vi "REPORT_GEAR_save_pdf.vi"(8 "error_in":errorcluster) -> (0 "error_out":errorcluster)   [LabVIEW 2019]
uses:
  FGV/REPORTS_records_display/FGV_REPORTS_records_display.ctl
  typedef/REPORT_GEAR_all_info.ctl
  typedef/REPORT_GEAR_header_data_display.ctl
  typedef/REPORT_GEAR_statuses.ctl
  <vilib>/Exaprom PDF/Controls/Page Controls/Page setup.ctl
  <vilib>/Exaprom PDF/Controls/Page Controls/Page size.ctl
  <vilib>/Exaprom PDF/Controls/Page Controls/Page Orientation.ctl
  <vilib>/Exaprom PDF/Controls/Page Controls/Page Layout Custom.ctl
  <vilib>/Exaprom PDF/Controls/Page Controls/Page margins.ctl
  <vilib>/Exaprom PDF/Controls/Image Controls/Image alignment and position.ctl
  <vilib>/Exaprom PDF/Controls/Image Controls/Image aligment.ctl
  <vilib>/Exaprom PDF/Controls/Table Controls/Row Predefined borders cluster.ctl
  <vilib>/Exaprom PDF/Controls/Table Controls/Row Predefined borders.ctl
  <vilib>/Exaprom PDF/Controls/Table Controls/Cell Font, type, Alignment and LS V2.ctl
  <vilib>/Exaprom PDF/Controls/Table Controls/Cell Type, Alignment and LS.ctl
  <vilib>/Exaprom PDF/Controls/Table Controls/Cell Alignment 20px.ctl
  <vilib>/Exaprom PDF/Controls/Table Controls/Text vertical arrangement.ctl
  <vilib>/Exaprom PDF/Controls/Text Controls/Line spacing.ctl
  <vilib>/Exaprom PDF/Controls/Font Controls/Font complete cluster.ctl
  <vilib>/Exaprom PDF/Controls/Font Controls/Font size.ctl
  <vilib>/Exaprom PDF/Controls/Font Controls/Font color.ctl
  <vilib>/Exaprom PDF/Controls/Font Controls/Type and encoding.ctl
  <vilib>/Exaprom PDF/Controls/Text Controls/Unicode/Type and run direction.ctl
  REPORT_font_for_pdf_report.ctl
  _misc/AULocalize/SubVIs/Get Localized Phrase Compact Interface 0D.vi
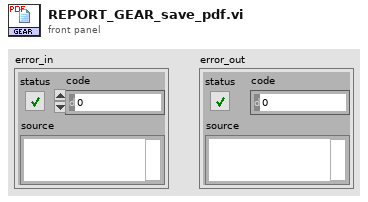
[diagram p1: front panel]
types:
  T1 = typedef "REPORT_GEAR_all_info.ctl" = cluster{"serial":string, "filter_OP":string, "REPORT_GEAR_header":T2, "operations":string[][], "operation_statuses":T3[], "results":string[][], "result_statuses":T3[], "batches":string[][], "batch_statuses":T3[], "column_headers":string[], "displayed_rows":string[][], "displayed_statuses":T3[], "column_widths":i16[]}
  T2 = typedef "REPORT_GEAR_header_data_display.ctl" = cluster{"ID":string, "creation_time":string, "last_station":string, "last_status":string, "pinion_serial":string, "batch_code":string}
  T3 = typedef "REPORT_GEAR_statuses.ctl" = enum16{"OP_OK_hide", "OP_OK_show", "OP_NOK_hide", "OP_NOK_show", "OP_interrupted_hide", "OP_interrupted_show", "OP_in_operation_hide", "OP_in_operation_show", "OP_unexpected_hide", "OP_unexpected_show", "RE_REAL_OK", "RE_REAL_NOK", "RE_STRING", "RE_sub_header", "RE_no_data", "RE_unexpected", "BA_sub_header", "BA_data", "BA_no_data"}
  T4 = typedef "FGV_REPORTS_records_display.ctl" = enum16{"initialize", "GEAR_set_serial", "GEAR_set_header", "GEAR_set_operations", "GEAR_set_results", "GEAR_set_batches", "GEAR_get_serial", "GEAR_get_operation_IDs", "GEAR_toggle_results", "GEAR_show_all_results", "GEAR_hide_all_results", "GEAR_display", "GEAR_filter", "GEAR_restore", "GEAR_clear", "GEAR_get_all_info", "DATES_set_dates", "DATES_set_gears", "DATES_display", "DATES_filter", "DATES_first_page", "DATES_previous_page", "DATES_next_page", "DATES_last_page", "DATES_restore", "DATES_clear", "DATES_get_all_info", "PBATCH_set_batch_no", "PBATCH_set_gears", "PBATCH_display", "PBATCH_filter", "PBATCH_first_page", "PBATCH_previous_page", "PBATCH_next_page", "PBATCH_last_page", "PBATCH_restore", "PBATCH_clear", "PBATCH_get_all_info", "OPRTN_set_OP", "OPRTN_set_dates", "OPRTN_set_gears", "OPRTN_set_hidden_columns", "OPRTN_display", "OPRTN_filter", "OPRTN_filter_no_page_reset", "OPRTN_first_page", "OPRTN_previous_page", "OPRTN_next_page", "OPRTN_last_page", "OPRTN_restore", "OPRTN_clear", "OPRTN_get_all_info", "CFG_set_type", "CFG_set_dates", "CFG_set_records", "CFG_display", "CFG_filter", "CFG_first_page", "CFG_previous_page", "CFG_next_page", "CFG_last_page", "CFG_restore", "CFG_clear", "CFG_get_all_info", "AUDIT_set_dates", "AUDIT_set_records", "AUDIT_display", "AUDIT_filter", "AUDIT_first_page", "AUDIT_previous_page", "AUDIT_next_page", "AUDIT_last_page", "AUDIT_restore", "AUDIT_clear", "AUDIT_get_all_info", "OKNOK_set_dates", "OKNOK_set_records", "OKNOK_display", "OKNOK_restore", "OKNOK_clear", "OKNOK_get_all_info", "REWORKS_set_dates", "REWORKS_set_from_to", "REWORKS_set_records", "REWORKS_display", "REWORKS_filter", "REWORKS_first_page", "REWORKS_previous_page", "REWORKS_next_page", "REWORKS_last_page", "REWORKS_restore", "REWORKS_clear", "REWORKS_get_all_info", "PACE_set_dates", "PACE_set_limits", "PACE_set_records", "PACE_display", "PACE_restore", "PACE_clear", "PACE_get_all_info", "CBATCH_set_code", "CBATCH_set_records", "CBATCH_display", "CBATCH_filter", "CBATCH_first_page", "CBATCH_previous_page", "CBATCH_next_page", "CBATCH_last_page", "CBATCH_restore", "CBATCH_clear", "CBATCH_get_all_info", "CMPNT_set_serial", "CMPNT_set_records", "CMPNT_display", "CMPNT_first_page", "CMPNT_previous_page", "CMPNT_next_page", "CMPNT_last_page", "CMPNT_restore", "CMPNT_clear", "CMPNT_get_all_info", "clear"}
  T5 = typedef "REPORT_font_for_pdf_report.ctl" = cluster{"Name":string, "Size":T6, "Color":T7, "Style":cluster{"Bold":bool, "Italic":bool, "Underline":bool, "Strikeout":bool}, "Type":T8}
  T6 = typedef "Font size.ctl" = sgl
  T7 = typedef "Font color.ctl" = u32
  T8 = typedef "Type and encoding.ctl" = cluster{"Type&direction":T9, "Embedded":bool, "Encoding":string}
  T9 = typedef "Type and run direction.ctl" = enum16{"Select", "ASCII", "UTF-16", "UTF-16 (default)", "UTF-16 (LTR)", "UTF-16 (RTL)"}
  T10 = typedef "Cell Font, type, Alignment and LS V2.ctl" = cluster{"Cell Type, Alignment and LS":T11, "Font":T15}
  T11 = typedef "Cell Type, Alignment and LS.ctl" = cluster{"Cell Alignment":T12, "Text rotation":T13, "Line spacing":T14}
  T12 = typedef "Cell Alignment 20px.ctl" = u16
  T13 = typedef "Text vertical arrangement.ctl" = enum16{"None", "Clockwise", "Counterclockwise"}
  T14 = typedef "Line spacing.ctl" = enum16{"Select", "1.0", "1.5", "2.0"}
  T15 = typedef "Font complete cluster.ctl" = cluster{"Name":string, "Size":T6, "Color":T7, "Style":cluster{"Bold":bool, "Italic":bool, "Underline":bool, "Strikeout":bool}, "Type":T8}
  T16 = typedef "Row Predefined borders cluster.ctl" = cluster{"Borders":T17, "Header":cluster{"Thickness":sgl, "Line":u32, "Background ":u32}, "Data":cluster{"Thickness":sgl, "Line":u32, "Background ":u32}}
  T17 = typedef "Row Predefined borders.ctl" = u16
  T18 = typedef "Image alignment and position.ctl" = cluster{"Alignment":T19, "X ":sgl, "Y":sgl, "Indentation":sgl}
  T19 = typedef "Image aligment.ctl" = enum16{"Absolute (X,Y)", "Left", "Center", "Right", "Left (textwrap)", "Right (textwrap)"}
  T20 = typedef "Page setup.ctl" = cluster{"Page Size":T21, "Orientation":T22, "Custom Size":T23, "Margins":T24}
  T21 = typedef "Page size.ctl" = i32
  T22 = typedef "Page Orientation.ctl" = enum16{"Portrait", "Landscape"}
  T23 = typedef "Page Layout Custom.ctl" = cluster{"Width":sgl, "Height":sgl}
  T24 = typedef "Page margins.ctl" = cluster{"Left":sgl, "Right":sgl, "Top":sgl, "Bottom":sgl}
  T25 = typedef "Table Appearance and Font Row [ ].ctl" = T26[]
  T26 = typedef "One Row Appearance.ctl" = cluster{"Row":T27, "Cell [ ]":T28[]}
  T27 = typedef "Row from to.ctl" = cluster{"From #":i16, "to #":i16}
  T28 = typedef "Cell, Alignment, LS and Font - hide Vmerge.ctl" = cluster{"Text":T11, "Cell Appearance":T29, "HMerge":T31, "VMerge":T32, "Font":T15}
  T29 = typedef "Cell Appearance.ctl" = cluster{"Border":T30, "Thickness":sgl, "Color":u32, "BG":u32}
  T30 = typedef "Cell Border 20 px.ctl" = u16
  T31 = typedef "Merge Horizontal.ctl" = cluster{"From":i8, "to":i8}
  T32 = typedef "Merge Vertical.ctl" = cluster{"From":i8, "to":i8}
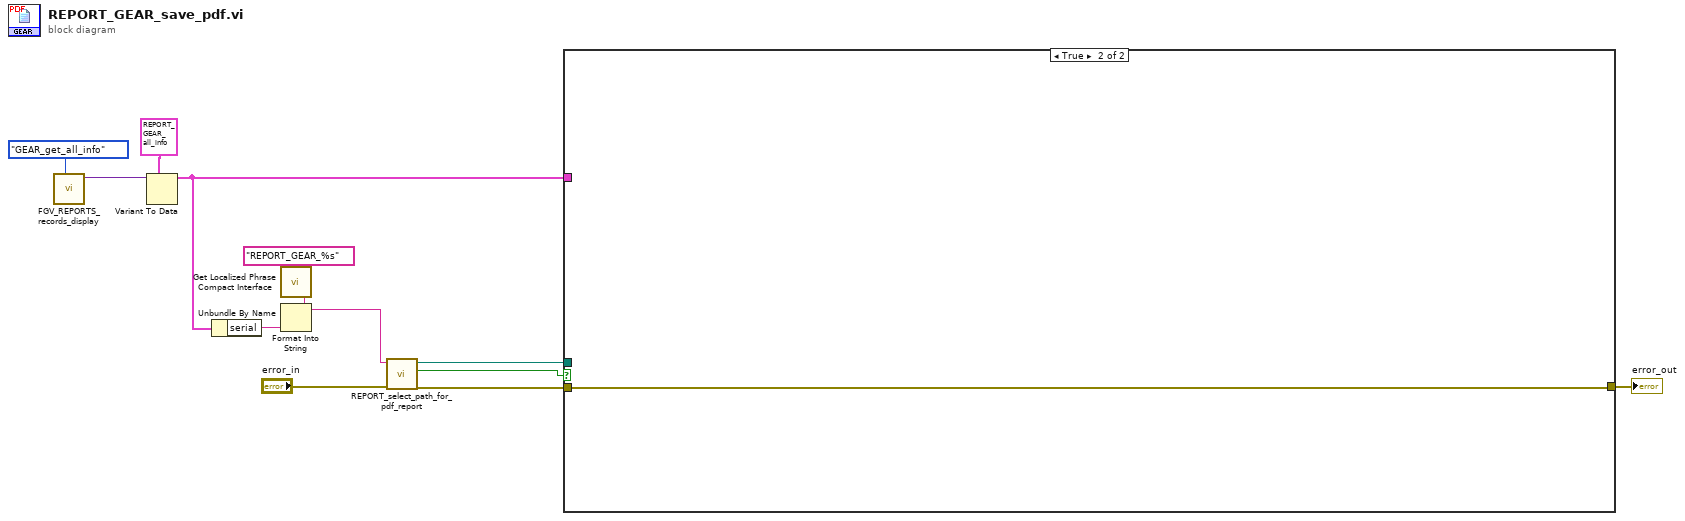
[diagram p0: block diagram]
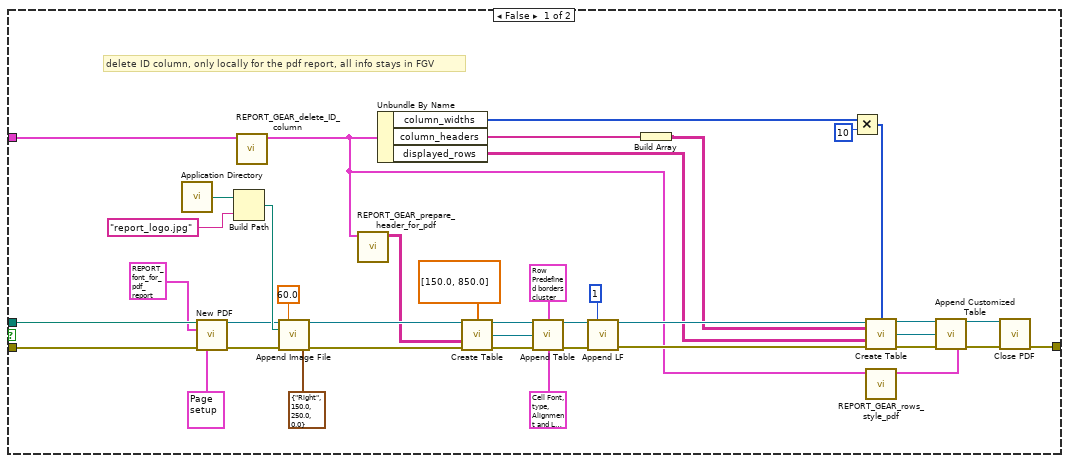
[diagram p2: hidden frame]
diagram:
  n1 = call "FGV_REPORTS_records_display.vi"("options"=FGV_REPORTS_records_display."GEAR_get_all_info") -> ("output"=w12:variant)  [unwired: 9 in, 1 out]
  n2 = Variant To Data(type=T1 {"serial"="", "filter_OP"="", "REPORT_GEAR_header"={"ID"="", "creation_time"="", "last_station"="", "last_status"="", "pinion_serial"="", "batch_code"=""}, "operations"=[], "operation_statuses"=[], "results"=[], "result_statuses"=[], "batches"=[], "batch_statuses"=[], "column_headers"=[], "displayed_rows"=[], "displayed_statuses"=[], "column_widths"=[]} ("REPORT_GEAR_all_info"), Variant=w12) -> (data=w3:T1)  [unwired: 1 in, 1 out]
  n3 = Unbundle By Name(w3) -> ("serial"=w5:string)
  n4 = call-poly "Get Localized Phrase Compact Interface.vi"("Key"="REPORT_GEAR_%s" ("report_title")) -> ("Translated Phrase"=w1:string)
  n5 = Format Into String(format string=w1, w5) -> (resulting string=w4:string)  [unwired: 2 in, 1 out]
  n6 = call "REPORT_select_path_for_pdf_report.vi"("error_in"="error_in", "report_title"=w4) -> ("error_out"=w7:errorcluster, "cancelled"=w2:bool, "path_to_report"=w8:path)  [unwired: 7 in]
  n7 = case shown="True" w2 {
    tunnel: [w53 w54] -> w9
    tunnel: w8 -> [w52 _]
    tunnel: w7 -> [w51 w54]
    tunnel: w3 -> [w17 _]
    frame False {
      # "delete ID column, only locally for the pdf report, all info stays in FGV"
      n8 = call <vilib>:"Application Directory.vi"() -> ("Application Directory"=w44:path)
      n9 = call <vilib>:"New PDF.vi"("PDF Path"=w52, "Default Font"=T5 {"Name"="Consolas", "Size"=10.0, "Color"=0, "Style"={"Bold"=FALSE, "Italic"=FALSE, "Underline"=FALSE, "Strikeout"=FALSE}, "Type"={"Type&direction"=enum."ASCII", "Embedded"=FALSE, "Encoding"="CP855"}}, "error in (no error)"=w51, "Page Setup"=T20 {"Page Size"=11, "Orientation"=enum."Landscape", "Custom Size"={"Width"=216.0, "Height"=279.0}, "Margins"={"Left"=10.0, "Right"=10.0, "Top"=10.0, "Bottom"=10.0}}) -> ("PDF Report"=w38:refnum<class "PDF Report Class.lvclass">, "error out"=w39:errorcluster)  [unwired: 7 in, 3 out]
      n10 = Build Path(base path=w44, name or relative path="report_logo.jpg") -> (appended path=w40:path)
      n11 = call "REPORT_GEAR_delete_ID_column.vi"("REPORT_GEAR_all_info"=w17) -> ("REPORT_GEAR_all_info_ID_deleted"=w16:T1)  [unwired: 10 in]
      n12 = call <vilib>:"Append Image File.vi"("PDF Report IN"=w38, "Scale (%)"=sgl 60.0, "Image path"=w40, "error in (no error)"=w39, "Position and indentation"=T18 {"Alignment"=enum."Right", "X "=150.0, "Y"=250.0, "Indentation"=0.0}) -> ("PDF Report OUT"=w19:refnum<class "PDF Report Class.lvclass">, "error out"=w18:errorcluster)  [unwired: 7 in, 2 out]
      n13 = call "REPORT_GEAR_prepare_header_for_pdf.vi"("REPORT_GEAR_all_info"=w16) -> ("report_header"=w14:string[][])  [unwired: 10 in]
      n14 = Unbundle By Name(w16) -> ("column_widths"=w15:i16[], "column_headers"=w31:string[], "displayed_rows"=w30:string[][])
      n15 = call <vilib>:"Create Table.vi"("PDF Report IN"=w19, "Table columnWidth [ ]"=sgl[] [150.0, 850.0], "Text Data 2D [ ]"=w14, "error in (no error)"=w18) -> ("PDF Report duplicate"=w27:refnum<class "PDF Report Class.lvclass">, "PDF Table"=w26:refnum<class "Pdfp Table Class.lvclass">, "error out"=w25:errorcluster)  [unwired: 9 in]
      n16 = call <vilib>:"Append Table.vi"("PDF Report IN"=w27, "Predefined Borders"=T16 {"Borders"=0, "Header"={"Thickness"=0.0, "Line"=0, "Background "=16777215}, "Data"={"Thickness"=0.0, "Line"=0, "Background "=16777215}}, "PDF Table"=w26, "error in (no error)"=w25, "Datas format"=T10 {"Cell Type, Alignment and LS"={"Cell Alignment"=0, "Text rotation"=enum."None", "Line spacing"=enum."Select"}, "Font"={"Name"="Consolas", "Size"=-1.0, "Color"=0, "Style"={"Bold"=FALSE, "Italic"=FALSE, "Underline"=FALSE, "Strikeout"=FALSE}, "Type"={"Type&direction"=enum."Select", "Embedded"=FALSE, "Encoding"=""}}}) -> ("PDF Report OUT"=w24:refnum<class "PDF Report Class.lvclass">, "error out"=w23:errorcluster)  [unwired: 9 in]
      n17 = call <vilib>:"Append LF.vi"("PDF Report IN"=w24, "Number of LF (default 1)"=u8 1, "error in (no error)"=w23) -> ("PDF Report duplicate"=w36:refnum<class "PDF Report Class.lvclass">, "error out"=w35:errorcluster)  [unwired: 11 in]
      n18 = Build Array(w31) -> (w32:string[][])
      n19 = Multiply(x=w15, y=i16 10) -> (x*y=w29:i16[])
      n20 = call <vilib>:"Create Table.vi"("PDF Report IN"=w36, "Table columnWidth [ ]"=w29, "Column Headers 2D [ ]"=w32, "Text Data 2D [ ]"=w30, "error in (no error)"=w35) -> ("PDF Report duplicate"=w33:refnum<class "PDF Report Class.lvclass">, "PDF Table"=w47:refnum<class "Pdfp Table Class.lvclass">, "error out"=w50:errorcluster)  [unwired: 8 in]
      n21 = call "REPORT_GEAR_rows_style_pdf.vi"("REPORT_GEAR_all_info"=w16) -> ("Row  [ ]"=w28:T25)  [unwired: 10 in]
      n22 = call <vilib>:"Append Customized Table.vi"("PDF Report IN"=w33, "PDF Table"=w47, "error in (no error)"=w50, "Row  [ ]"=w28) -> ("PDF Report OUT"=w48:refnum<class "PDF Report Class.lvclass">, "error out"=w49:errorcluster)  [unwired: 10 in]
      n23 = call <vilib>:"Close PDF.vi"("PDF Report"=w48, "error in (no error)"=w49) -> ("error out"=w53:errorcluster)  [unwired: 12 in, 1 out]
    }
    frame True {
    }
  }
  "error_out" <- w9
